vi "StashInactivePrefSets.vi"(8 "error in (no error)":errorcluster, 9 "Active PrefSet":string, 10 "node in":refnum<k20>, 11 "Preferences in":refnum<class "SetListPrefs.lvclass">) -> (0 "error out":errorcluster, 2 "node out":refnum<k20>, 3 "Preferences out":refnum<class "SetListPrefs.lvclass">)   [LabVIEW 2013, in "SetListPrefs.lvclass"]
uses:
  SetListPrefs.lvclass
  <vilib>/Utility/error.llb/DialogType.ctl
  SetListPrefs.lvclass/SetListPrefs.ctl
  <vilib>/xml/Close Reference(Node).vi
  <vilib>/xml/NI_XML.lvlib
  <resource>/objmgr/DOMUserDefRef.rc
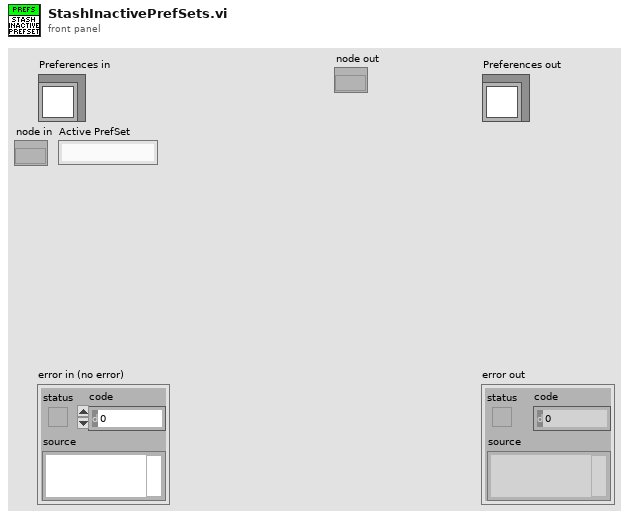
[diagram p1: front panel]
types:
  T1 = typedef "DialogType.ctl" = u16
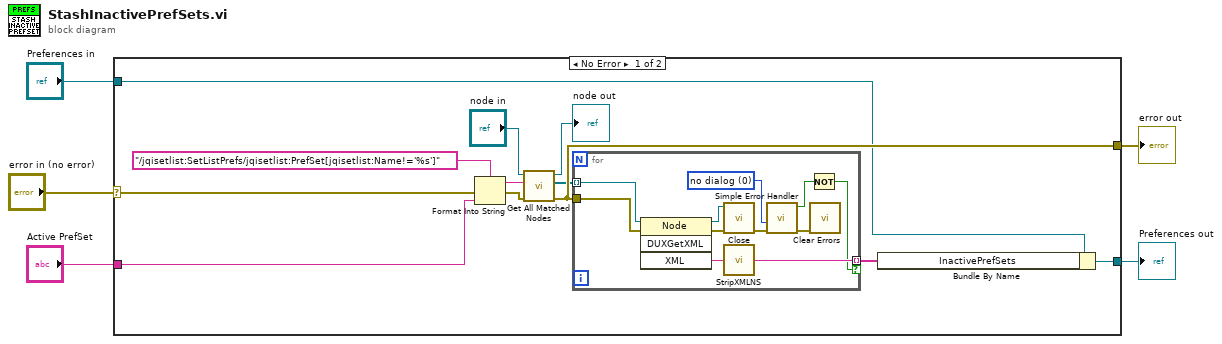
[diagram p0: block diagram]
diagram:
  n1 = case shown="No Error" "error in (no error)" {
    selector: "error in (no error)" -> [w15 w30]
    tunnel: [w12 w30] -> w4
    tunnel: [w6 w29] -> w2
    tunnel: "Preferences in" -> [w7 w29]
    tunnel: "Active PrefSet" -> [w8 _]
    frame No Error {
      n2 = Format Into String(format string="/jqisetlist:SetListPrefs/jqisetlist:PrefSet[jqisetlist:Name!='%s']" ("XPath expression"), error in=w15, w8) -> (resulting string=w14:string, error out=w13:errorcluster)  [unwired: 1 in]
      n3 = call <vilib>:"Get All Matched Nodes.vi"("error in (no error)"=w13, "XPath expression"=w14, "node in"="node in") -> ("error out"=w12:errorcluster, "node result array"=w11:refnum<k20>[], "node out"=→"node out":refnum<k20>)  [unwired: 6 in]
      n4 = for {
        tunnel: [w25] -> w17 mode=indexing if=w18
        tunnel: w12 -> [w24]
        tunnel: w11 -> [w23] mode=indexing
        w21 = T1 0 items=["no dialog", "OK message", "continue or stop message", "OK message + warnings", "continue/stop + warnings"] ("type of dialog (OK msg:1)")
        n5 = invoke class="Node" method="DUXGetXML"(reference=w23, error in=w24) -> (reference out=w28:refnum<k20>, error out=w27:errorcluster, "XML"=w26:string)  [unwired: 2 in, 1 out]
        n6 = call-poly <vilib>:"Close.vi"("error in (no error)"=w27, "node"=w28) -> ("error out"=w22:errorcluster)  [unwired: 7 in]
        n7 = call "StripXMLNS.vi"("XML in"=w26) -> ("XML out"=w25:string)
        n8 = call <vilib>:"Simple Error Handler.vi"("type of dialog (OK msg:1)"=w21, "error in (no error)"=w22) -> ("error?"=w19:bool, "error out"=w20:errorcluster)  [unwired: 3 in, 3 out]
        n9 = Not(x=w19) -> (.not. x?=w18:bool)
        n10 = call <vilib>:"Clear Errors.vi"("error in (no error)"=w20) -> ()  [unwired: 6 in, 1 out]
      }
      n11 = Bundle By Name(cluster=w7, "InactivePrefSets"=w17) -> (w6:refnum<class "SetListPrefs.lvclass">)
    }
    frame Error {
    }
  }
  "error out" <- w4
  "Preferences out" <- w2
